vi "PantherLAB Branding.vi"(8 "error in":errorcluster, 11 "This VI":refnum<vi>) -> ()   [LabVIEW 2016, in "PantherLAB_Scripting.lvlib"]
uses:
  <vilib>/Utility/miscctls.llb/LVRowAndColumnTypeDef.ctl
  PantherLAB_Scripting.lvlib
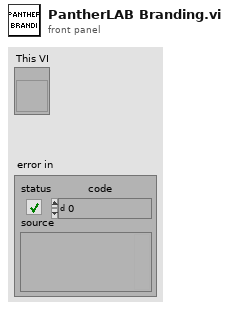
[diagram p1: front panel]
types:
  T1 = cluster{"Gris Obscuro Azul":u32, "Gris Medio Azul":u32, "Gris Claro Azul":u32, "Amarillo":u32, "Text color":u32, "Transparent":u32, "Fuente":string, "Text.Font:Size":u32}
  T2 = typedef "LVRowAndColumnTypeDef.ctl" = cluster{"Row":i32, "Column":i32}
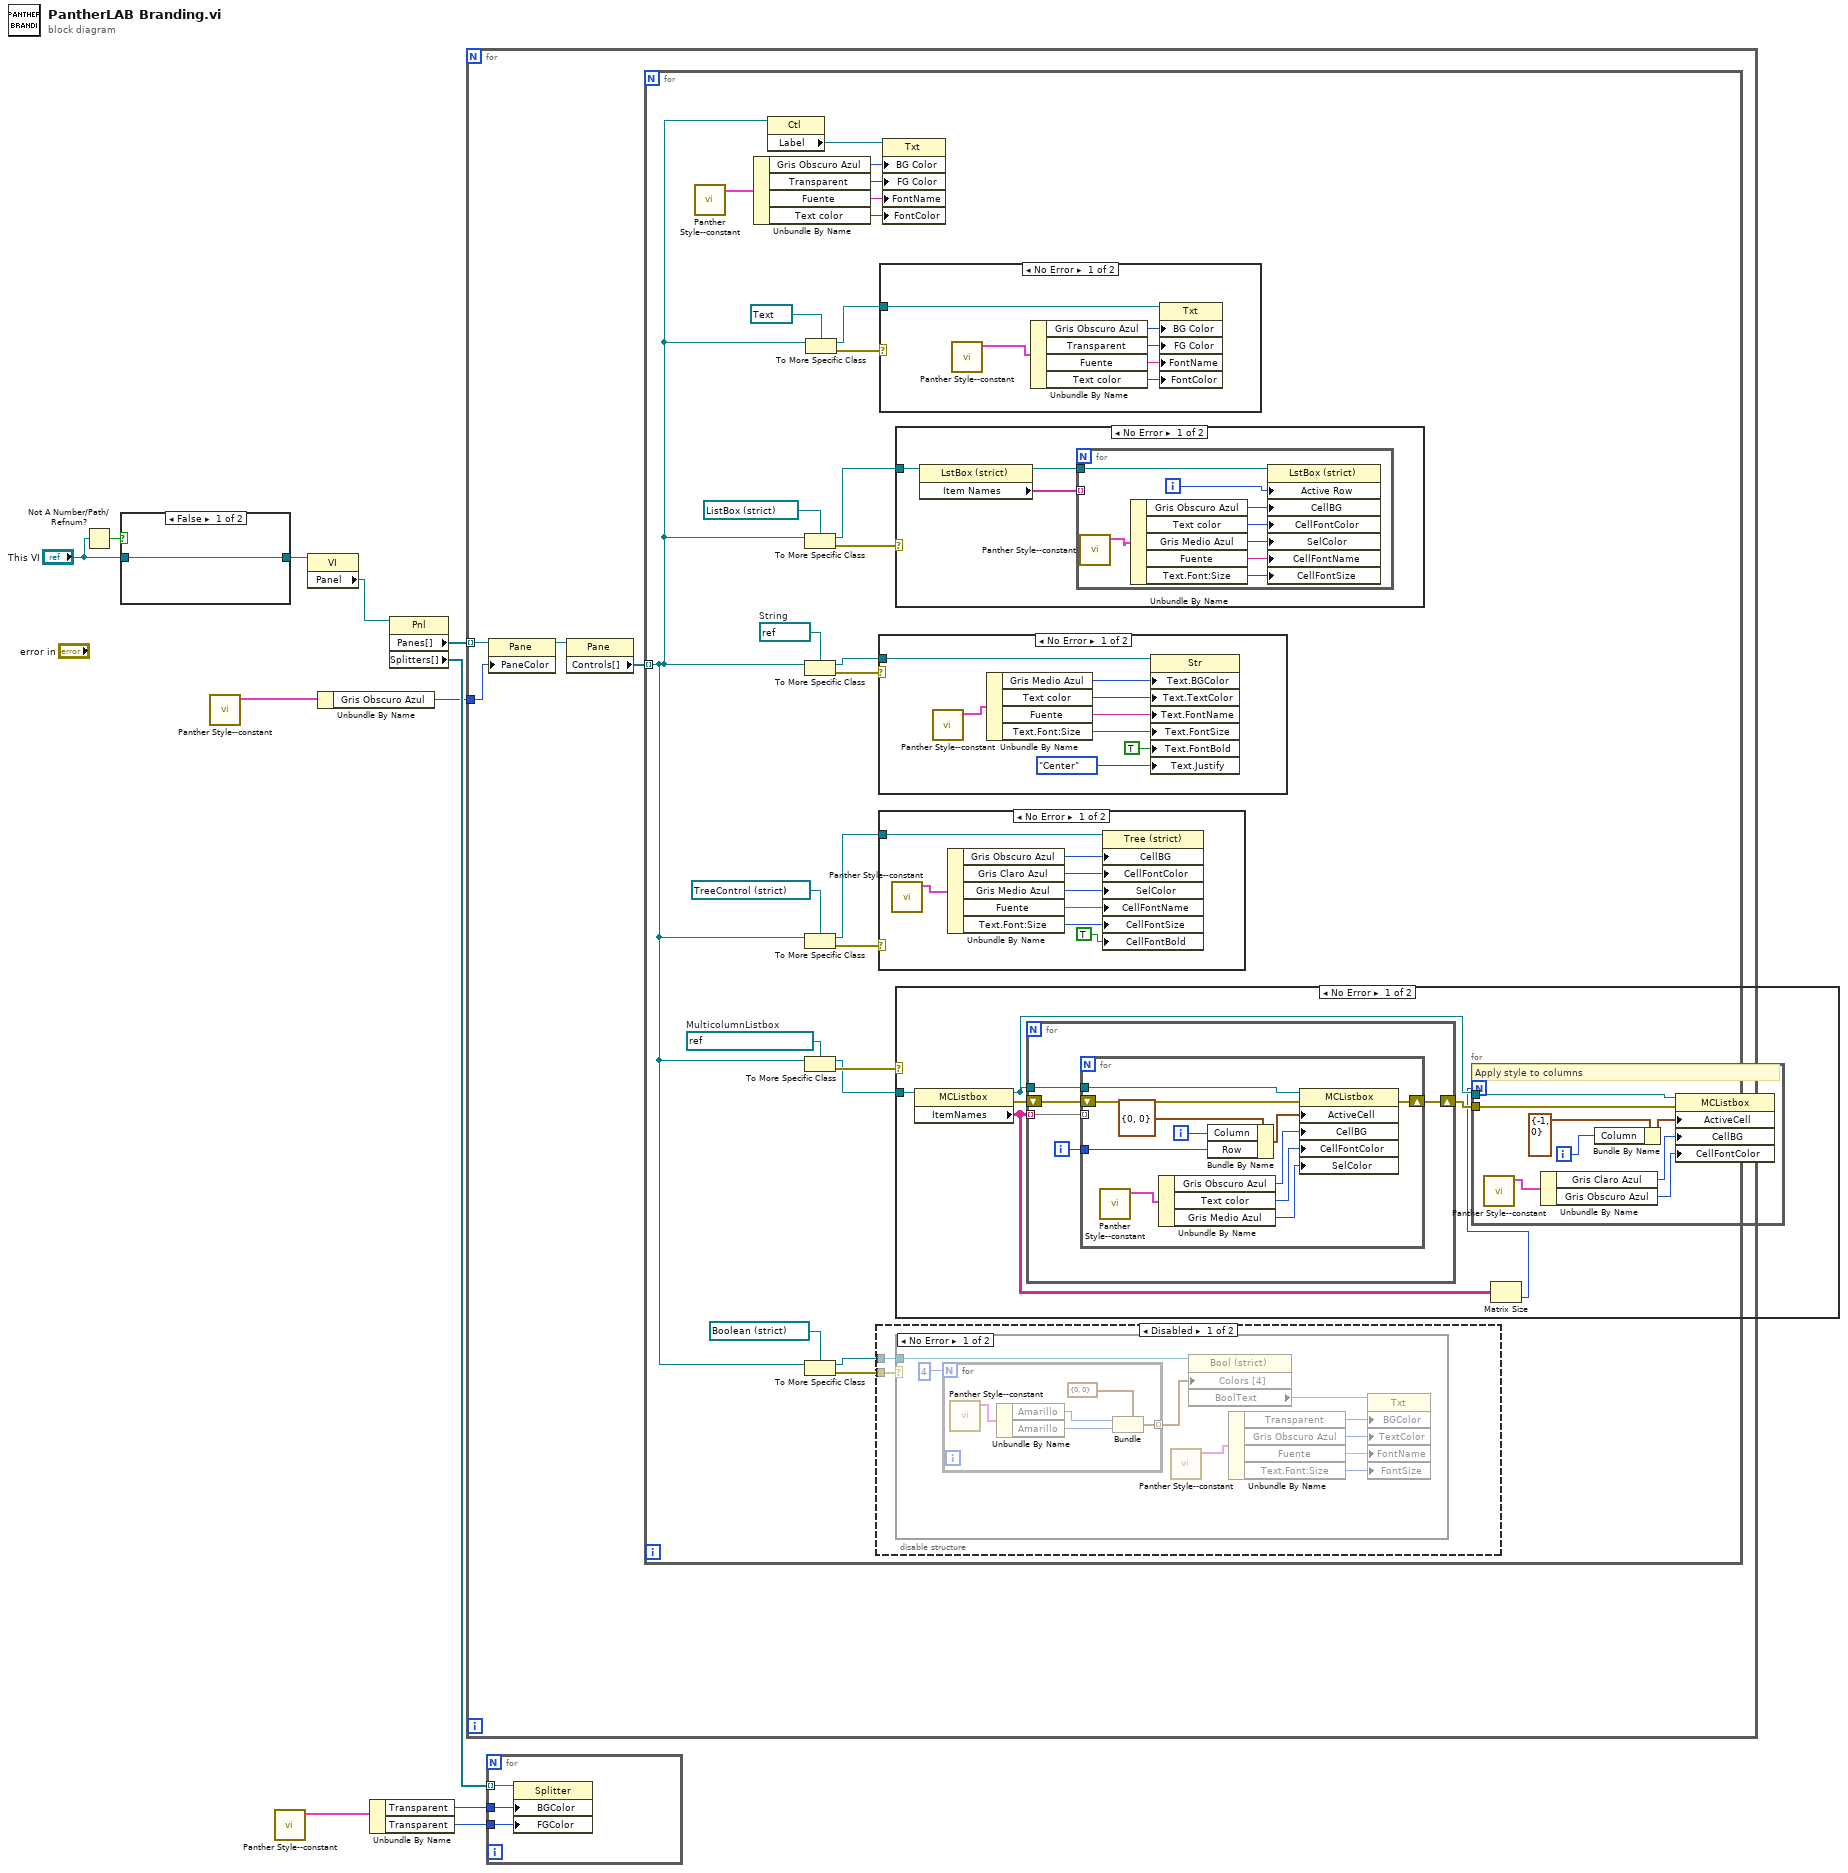
[diagram p0: block diagram]
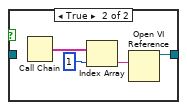
[diagram p9: hidden frame]
diagram:
  n1 = Not A Number/Path/Refnum?(number/path/refnum="This VI") -> (NaN/Path/Refnum?=w11:bool)
  n2 = case shown="False" w11 {
    tunnel: [w12 w13] -> w9
    tunnel: "This VI" -> [w12 _]
    frame False {
    }
    frame True {
      n3 = Call Chain() -> (call chain=w16:string[])
      n4 = Index Array(array=w16, index=1) -> (element=w14:string)
      n5 = Open VI Reference(vi path=w14) -> (vi reference=w13:refnum<vi>)  [unwired: 5 in, 1 out]
    }
  }
  n6 = call "Panther Style--constant.vi"() -> ("Style"=w2:T1)  [unwired: 11 in]
  n7 = call "Panther Style--constant.vi"() -> ("Style"=w1:T1)  [unwired: 11 in]
  n8 = property class="VI"(reference=w9) -> ("Panel"=w8:refnum<vi>)  [unwired: 1 in, 2 out]
  n9 = Unbundle By Name(w2) -> ("Gris Obscuro Azul"=w3:u32)
  n10 = Unbundle By Name(w1) -> ("Transparent"=w5:u32, "Transparent"=w4:u32)
  n11 = property class="Pnl"(reference=w8) -> ("Panes[]"=w7:refnum<vi>[], "Splitters[]"=w6:refnum<vi>[])  [unwired: 1 in, 2 out]
  n12 = for {
    tunnel: w7 -> [w20] mode=indexing
    tunnel: w3 -> [w17]
    n13 = property class="Pane"(reference=w20, "PaneColor"=w17) -> (reference out=w19:refnum<vi>)  [unwired: 1 in, 1 out]
    n14 = property class="Pane"(reference=w19) -> ("Controls[]"=w18:refnum<vi>[])  [unwired: 1 in, 2 out]
    n15 = for {
      tunnel: w18 -> [w21] mode=indexing
      w34 = refnum<vi> refnum  # String
      w35 = refnum<vi> refnum  # MulticolumnListbox
      n16 = call "Panther Style--constant.vi"() -> ("Style"=w22:T1)  [unwired: 11 in]
      n17 = Unbundle By Name(w22) -> ("Gris Obscuro Azul"=w31:u32, "Transparent"=w28:u32, "Fuente"=w30:string, "Text color"=w29:u32)
      n18 = property class="Ctl"(reference=w21) -> ("Label"=w32:refnum<vi>)  [unwired: 1 in, 2 out]
      n19 = To More Specific Class(target class=refnum<vi> refnum ("Project history"), reference=w21) -> (specific class reference=w37:refnum<vi>, error out=w43:errorcluster)  [unwired: 1 in]
      n20 = To More Specific Class(target class=w34, reference=w21) -> (specific class reference=w33:refnum<vi>, error out=w41:errorcluster)  [unwired: 1 in]
      n21 = To More Specific Class(target class=refnum<vi> refnum ("Tree Control"), reference=w21) -> (specific class reference=w38:refnum<vi>, error out=w44:errorcluster)  [unwired: 1 in]
      n22 = To More Specific Class(target class=w35, reference=w21) -> (specific class reference=w36:refnum<vi>, error out=w42:errorcluster)  [unwired: 1 in]
      n23 = To More Specific Class(target class=refnum<vi> refnum ("Scan All"), reference=w21) -> (specific class reference=w39:refnum<vi>, error out=w45:errorcluster)  [unwired: 1 in]
      n24 = To More Specific Class(target class=refnum<vi> refnum ("Project history"), reference=w21) -> (specific class reference=w24:refnum<vi>, error out=w40:errorcluster)  [unwired: 1 in]
      n25 = disable-structure shown="Disabled" {
        disable-tunnel: w45 -> [w47 _]
        disable-tunnel: w39 -> [w46 _]
        frame Disabled {
          n26 = case shown="No Error" w47 {
            tunnel: w46 -> [w51 _]
            frame No Error {
              n27 = for {
                N: 4 -> [_]
                tunnel: [w60] -> w55 mode=indexing
                n28 = call "Panther Style--constant.vi"() -> ("Style"=w57:T1)  [unwired: 11 in]
                n29 = Unbundle By Name(w57) -> ("Amarillo"=w58:u32, "Amarillo"=w59:u32)
                n30 = Bundle(cluster=cluster{u32, u32} {0, 0} ("Colors [4]"), w58, w59) -> (w60:cluster{u32, u32})
              }
              n31 = call "Panther Style--constant.vi"() -> ("Style"=w48:T1)  [unwired: 11 in]
              n32 = property class="Bool (strict)"(reference=w51, "Colors [4]"=w55) -> ("BoolText"=w56:refnum<vi>)  [unwired: 1 in, 2 out]
              n33 = Unbundle By Name(w48) -> ("Transparent"=w53:u32, "Gris Obscuro Azul"=w52:u32, "Fuente"=w50:string, "Text.Font:Size"=w49:u32)
              n34 = property class="Txt"(reference=w56, "BGColor"=w53, "TextColor"=w52, "FontName"=w50, "FontSize"=w49) -> ()  [unwired: 1 in, 2 out]
            }
            frame Error {
            }
          }
        }
        frame Enabled {
        }
      }
      n35 = case shown="No Error" w41 {
        tunnel: w33 -> [w75 _]
        frame No Error {
          n36 = call "Panther Style--constant.vi"() -> ("Style"=w68:T1)  [unwired: 11 in]
          n37 = Unbundle By Name(w68) -> ("Gris Medio Azul"=w74:u32, "Text color"=w73:u32, "Fuente"=w72:string, "Text.Font:Size"=w71:u32)
          n38 = property class="Str"(reference=w75, "Text.BGColor"=w74, "Text.TextColor"=w73, "Text.FontName"=w72, "Text.FontSize"=w71, "Text.FontBold"=TRUE ("Text.Font:Bold"), "Text.Justify"=enum16{"Left", "Center", "Right"}."Center" ("Text.Justification")) -> ()  [unwired: 1 in, 2 out]
        }
        frame Error {
        }
      }
      n39 = case shown="No Error" w44 {
        tunnel: w38 -> [w109 _]
        frame No Error {
          n40 = call "Panther Style--constant.vi"() -> ("Style"=w106:T1)  [unwired: 11 in]
          n41 = Unbundle By Name(w106) -> ("Gris Obscuro Azul"=w113:u32, "Gris Claro Azul"=w112:u32, "Gris Medio Azul"=w111:u32, "Fuente"=w110:string, "Text.Font:Size"=w108:u32)
          n42 = property class="Tree (strict)"(reference=w109, "CellBG"=w113, "CellFontColor"=w112, "SelColor"=w111, "CellFontName"=w110, "CellFontSize"=w108, "CellFontBold"=TRUE ("Active Cell:Cell Font:Bold")) -> ()  [unwired: 1 in, 2 out]
        }
        frame Error {
        }
      }
      n43 = case shown="No Error" w40 {
        tunnel: w24 -> [w63 _]
        frame No Error {
          n44 = call "Panther Style--constant.vi"() -> ("Style"=w62:T1)  [unwired: 11 in]
          n45 = Unbundle By Name(w62) -> ("Gris Obscuro Azul"=w67:u32, "Transparent"=w64:u32, "Fuente"=w66:string, "Text color"=w65:u32)
          n46 = property class="Txt"(reference=w63, "BG Color"=w67, "FG Color"=w64, "FontName"=w66, "FontColor"=w65) -> ()  [unwired: 1 in, 2 out]
        }
        frame Error {
        }
      }
      n47 = property class="Txt"(reference=w32, "BG Color"=w31, "FG Color"=w28, "FontName"=w30, "FontColor"=w29) -> ()  [unwired: 1 in, 2 out]
      n48 = case shown="No Error" w43 {
        tunnel: w37 -> [w116 _]
        frame No Error {
          n49 = property class="LstBox (strict)"(reference=w116) -> (reference out=w115:refnum<vi>, "Item Names"=w114:string[])  [unwired: 1 in, 1 out]
          n50 = for {
            tunnel: w115 -> [w120]
            tunnel: w114 -> [_] mode=indexing
            i -> [w118]
            n51 = call "Panther Style--constant.vi"() -> ("Style"=w117:T1)  [unwired: 11 in]
            n52 = Unbundle By Name(w117) -> ("Gris Obscuro Azul"=w119:u32, "Text color"=w124:u32, "Gris Medio Azul"=w123:u32, "Fuente"=w122:string, "Text.Font:Size"=w121:u32)
            n53 = property class="LstBox (strict)"(reference=w120, "Active Row"=w118, "CellBG"=w119, "CellFontColor"=w124, "SelColor"=w123, "CellFontName"=w122, "CellFontSize"=w121) -> ()  [unwired: 1 in, 2 out]
          }
        }
        frame Error {
        }
      }
      n54 = case shown="No Error" w42 {
        tunnel: w36 -> [w79 _]
        frame No Error {
          n55 = property class="MCListbox"(reference=w79) -> (reference out=w78:refnum<vi>, error out=w81:errorcluster, "ItemNames"=w77:string[][])  [unwired: 1 in]
          n56 = for {
            tunnel: w78 -> [w92]
            tunnel: w77 -> [w90] mode=indexing
            shift-right: [w93] -> w80
            shift-left: w81 -> [w94]
            i -> [w91]
            n57 = for {
              tunnel: w92 -> [w101]
              tunnel: w91 -> [w96]
              tunnel: w90 -> [_] mode=indexing
              shift-right: [w104] -> w93
              shift-left: w94 -> [w105]
              i -> [w97]
              n58 = call "Panther Style--constant.vi"() -> ("Style"=w95:T1)  [unwired: 11 in]
              n59 = Unbundle By Name(w95) -> ("Gris Obscuro Azul"=w100:u32, "Text color"=w103:u32, "Gris Medio Azul"=w102:u32)
              n60 = Bundle By Name(cluster=T2 {"Row"=0, "Column"=0} ("Active Cell:Active Cell"), "Column"=w97, "Row"=w96) -> (w98:T2)
              n61 = property class="MCListbox"(reference=w101, error in=w105, "ActiveCell"=w98, "CellBG"=w100, "CellFontColor"=w103, "SelColor"=w102) -> (error out=w104:errorcluster)  [unwired: 1 out]
            }
          }
          n62 = Matrix Size(0:w77) -> (2:w76:i32)  [unwired: 1 out]
          n63 = for {
            N: w76 -> [_]
            tunnel: w80 -> [w89]
            tunnel: w78 -> [w88]
            i -> [w83]
            # "Apply style to columns"
            n64 = call "Panther Style--constant.vi"() -> ("Style"=w82:T1)  [unwired: 11 in]
            n65 = Unbundle By Name(w82) -> ("Gris Claro Azul"=w86:u32, "Gris Obscuro Azul"=w85:u32)
            n66 = Bundle By Name(cluster=T2 {"Row"=-1, "Column"=0} ("Active Cell:Active Cell"), "Column"=w83) -> (w84:T2)
            n67 = property class="MCListbox"(reference=w88, error in=w89, "ActiveCell"=w84, "CellBG"=w86, "CellFontColor"=w85) -> ()  [unwired: 2 out]
          }
        }
        frame Error {
        }
      }
    }
  }
  n68 = for {
    tunnel: w6 -> [w127] mode=indexing
    tunnel: w5 -> [w126]
    tunnel: w4 -> [w125]
    n69 = property class="Splitter"(reference=w127, "BGColor"=w126, "FGColor"=w125) -> ()  [unwired: 1 in, 2 out]
  }
